vi "Board Coordinate to Picture Rectangle.vi"(1 "Particle Size":u32, 2 "Coordinate":T2) -> (0 "rect":T1)   [LabVIEW 2019]
uses:
  Coordinate STYP.ctl
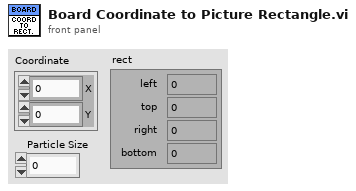
[diagram p1: front panel]
types:
  T1 = cluster{"left":i16, "top":i16, "right":i16, "bottom":i16}
  T2 = typedef "Coordinate STYP.ctl" = cluster{"X":i32, "Y":i32}
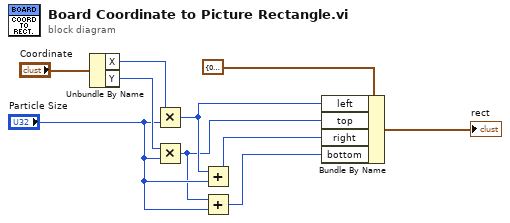
[diagram p0: block diagram]
diagram:
  n1 = Unbundle By Name("Coordinate") -> ("X"=w9:i32, "Y"=w8:i32)
  n2 = Multiply(x=w9, y="Particle Size") -> (x*y=w4:u32)
  n3 = Multiply(x=w8, y="Particle Size") -> (x*y=w3:u32)
  n4 = Add(x=w4, y="Particle Size") -> (x+y=w2:u32)
  n5 = Add(x=w3, y="Particle Size") -> (x+y=w1:u32)
  n6 = Bundle By Name(cluster=T1 {"left"=0, "top"=0, "right"=0, "bottom"=0} ("rect"), "left"=w4, "top"=w3, "right"=w2, "bottom"=w1) -> (→"rect":T1)
